vi "CRYGet Jump No and Name.vi"(5 "Jump No":i32) -> (4 "Active Cell String1":string, 6 "Active Cell String0":string)   [LabVIEW 2013]
uses:
  CRYProject Editor Global.vi
panel:
  in  "Temp No":i32
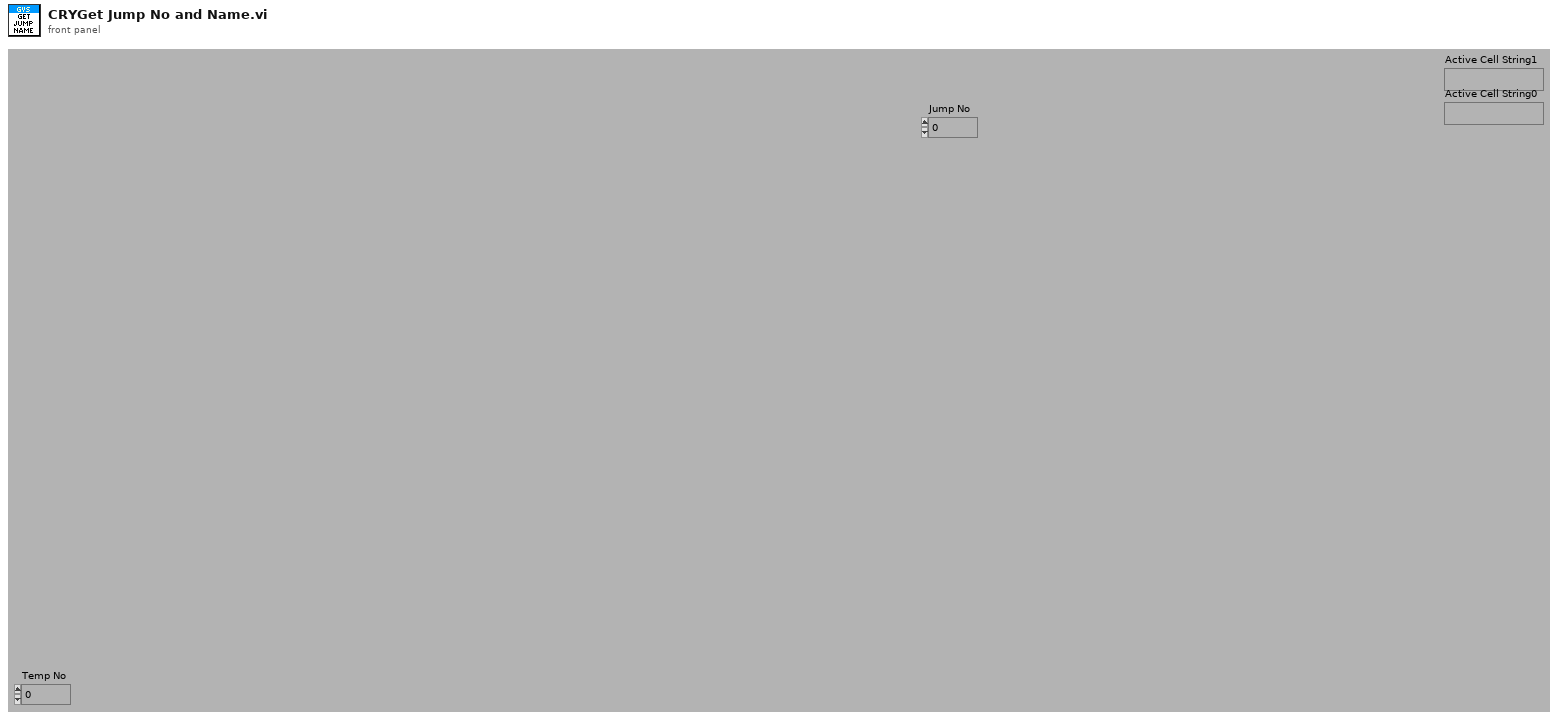
[diagram p1: front panel]
types:
  T1 = typedef "CRYTS.ctl" = cluster{"No.TS":u16, "TS File Path":path, "TS Name":string, "EditStepName":string, "Steps":T2[], "New State":bool, "Change State":bool, "Flattened CurveLib Data":string, "Document Data":string, "EditStepNo":u16, "Operator Start File":string, "Sequence Type":string, "Sequence Language":string}
  T2 = typedef "CRYStep.ctl" = cluster{"No.VI":i32, "Category":string, "StepName":string, "Seq setup flattened":string, "Comment":string, "Steps config.":bool[], "Jump config":i32[], "Start":dbl, "Increment":dbl, "Name":string, "Unit":string, "Y data":u16, "Y prefix":string, "Y dB ref":dbl, "Y unit":string, "Repeat State Array":cluster{"Start":dbl, "Increment":dbl, "Count":i32, "Num":i32}[]}
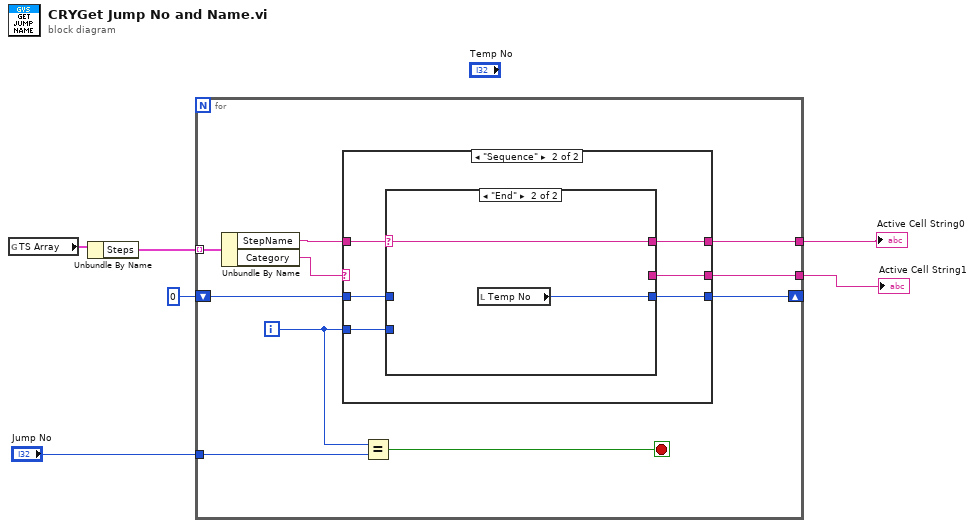
[diagram p0: block diagram]
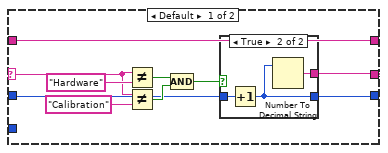
[diagram p2: hidden frame]
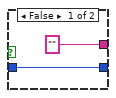
[diagram p3: hidden frame]
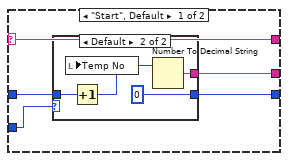
[diagram p4: hidden frame]
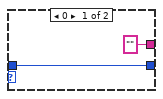
[diagram p5: hidden frame]
diagram:
  n1 = global read "CRYProject Editor Global.vi" "TS Array"() -> (w6:T1)
  n2 = Unbundle By Name(w6) -> ("Steps"=w5:T2[])
  n3 = for {
    shift-right: [w15] -> _
    shift-left: 0 ("Temp No") -> [w16]
    tunnel: w5 -> [w13] mode=indexing
    tunnel: "Jump No" -> [w10]
    tunnel: [w8] -> w1
    tunnel: [w7] -> w2
    i -> [w11]
    stop <- w9 stop-if-true
    n4 = Unbundle By Name(w13) -> ("StepName"=w12:string, "Category"=w14:string)
    n5 = case shown="\"Sequence\"" w14 {
      selector: w14 -> [w25 _]
      tunnel: w12 -> [w17 w37]
      tunnel: w11 -> [_ w36]
      tunnel: w16 -> [w20 w35]
      tunnel: [w19 w34] -> w15
      tunnel: [w18 w33] -> w8
      tunnel: [w17 w32] -> w7
      frame Default {
        n6 = Not Equal?(x=w25, y="Hardware" ("Down Step Name")) -> (x != y?=w23:bool)
        n7 = Not Equal?(x=w25, y="Calibration" ("Down Step Name")) -> (x != y?=w22:bool)
        n8 = Compound Arithmetic op=AND(w23, w22) -> (w21:bool)
        n9 = case shown="True" w21 {
          tunnel: w20 -> [w27 w31]
          tunnel: [w27 w30] -> w19
          tunnel: ["" w29] -> w18
          frame False {
          }
          frame True {
            n10 = Increment(x=w31) -> (x+1=w30:i32)
            n11 = Number To Decimal String(number=w30) -> (decimal integer string=w29:string)  [unwired: 1 in]
          }
        }
      }
      frame "Sequence" {
        n12 = case shown="\"End\"" w37 {
          selector: w37 -> [w38 w49]
          tunnel: w36 -> [w42 _]
          tunnel: w35 -> [w41 _]
          tunnel: [w40 w50] -> w34
          tunnel: [w39 _] -> w33
          tunnel: [w38 w49] -> w32
          frame "Start", Default {
            n13 = case shown="Default" w42 {
              tunnel: w41 -> [w44 w47]
              tunnel: [w44 0 ("Glyph Index")] -> w40
              tunnel: ["" w45] -> w39
              frame 0 {
              }
              frame Default {
                n14 = Increment(x=w47) -> (x+1=w46:i32)
                n15 = local write "Temp No"(w46) -> ()
                n16 = Number To Decimal String(number=w46) -> (decimal integer string=w45:string)  [unwired: 1 in]
              }
            }
          }
          frame "End" {
            n17 = local read "Temp No"() -> (w50:i32)
          }
        }
      }
    }
    n18 = Equal?(x=w11, y=w10) -> (x = y?=w9:bool)
  }
  "Active Cell String1" <- w1
  "Active Cell String0" <- w2
